vi "Build Weighted Array Histogram.vi"(4 "Reject Negative Weights (T)":bool=TRUE, 5 "Weights":dbl[](array[numeric]), 6 "Data Type (Plot Y Axis)":T4, 7 "Graph Caption (or Label) Text":string, 8 "error in (no error)":errorcluster, 9 "Histogram Options":T1 {"Max Histogram Size" format="%.0e"}, 10 "Plot/Dataset Name":string, 11 "Array":dbl[](array[numeric])) -> (0 "error out":errorcluster, 1 "Message":string, 3 "Data Statistics":dbl[](array[numeric]))   [LabVIEW 2021, in "Histogram Window.lvlib"]
uses:
  Histogram Window.lvlib
  Graphs/Plot Style 3.ctl
  Graphs/Graphs.lvlib
  Plot Histogram.ctl
  Histogram Data Statistics.ctl
  Histogram Window.vi
  Utilities/Utilities.lvlib
  Histogram Window Q Action v2.ctl
  Histogram Window Q Element v2.ctl
  8d0d2780-fcbe-40f9-8a45-ac027e873698.vi
  <userlib>/_OpenG.lib/array/array.llb/openg_array.lvlib
  <userlib>/_OpenG.lib/array/array.llb/Delete Elements from 1D Array (DBL)__ogtk.vi
  <userlib>/_OpenG.lib/array/array.llb/Filter 1D Array (DBL)__ogtk.vi
  Histogram Bin Position.ctl
  Histogram Bin Option.ctl
  Linear Histogram Options.ctl
  Source Data Type.ctl
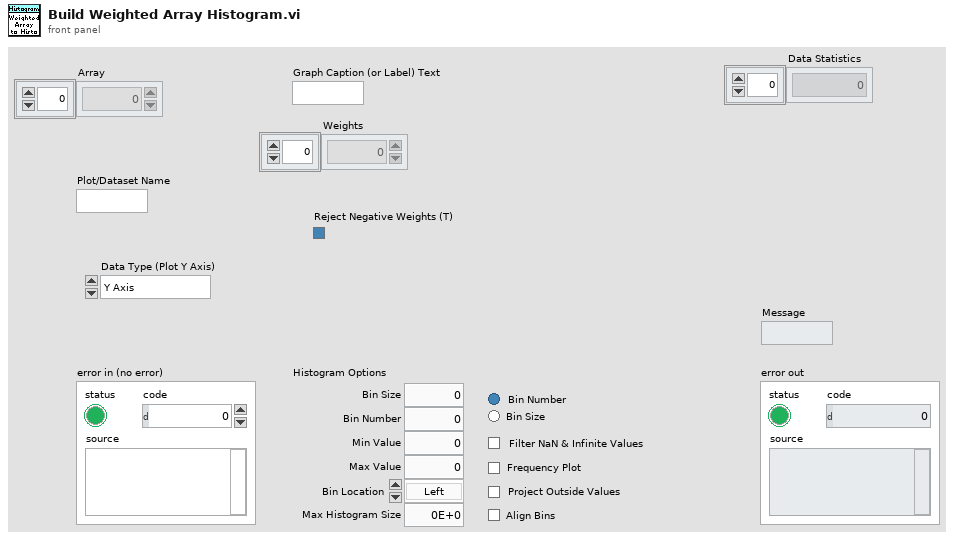
[diagram p1: front panel]
types:
  T1 = typedef "Histogram Window.lvlib/Linear Histogram Options.ctl" = cluster{"Bin Size":dbl, "Bin Number":i32, "Bin Option":T2, "Min Value":dbl, "Max Value":dbl, "Filter NaN & Infinite Values":bool, "Frequency Plot":bool, "Align Bins":bool, "Bin Location":T3, "Project Outside Values":bool, "Max Histogram Size":i32}
  T2 = typedef "Histogram Window.lvlib/Histogram Bin Option.ctl" = enum32{"Bin Number", "Bin Size"}
  T3 = typedef "Histogram Window.lvlib/Histogram Bin Position.ctl" = enum16{"Left", "Center", "Right"}
  T4 = typedef "Histogram Window.lvlib/Source Data Type.ctl" = enum16{"Y Axis", "X Axis", "Single Array"}
  T5 = typedef "Graphs.lvlib/Plot Style 3.ctl" = cluster{"Plot Style":enum16{"unchanged", "Line", "Symbol", "Line + Symbol", "Histogram", "Histogram + Symbol"}, "Histogram Type":enum16{"unchanged", "Left Bound", "Center", "Right Bound"}, "Line Tickness":enum16{"unchanged", "Thin", "1 pixel", "2 pixel", "3 pixel", "4 pixel", "5 pixel"}, "Line Style":enum16{"unchanged", "Plain", "Long Dash", "Short Dash", "Long-Short Dash", "Long-Short-Short Dash"}, "Point Style":enum16{"unchanged", "None", "Empty Circle", "Filled Circle", "Thick Circle", "Dotted Circle", "Empty Square", "Filled Square", "Thick Square", "Dotted Square", "Small Filled Square", "Dot", "Cross", "Tiny Cross", "Large X", "Small x", "Diamond", "Small Empty Square"}, "Line Color":u32, "Point Color":u32, "Anti-aliased":bool, "Line Color Chooser":enum16{"unchanged", "Color Box", "Color List"}, "Point Color Chooser":enum16{"unchanged", "Color Box", "Color List"}, "Line Color List":string, "Point Color List":string}
  T6 = typedef "Histogram Window.lvlib/Histogram Window Q Element v2.ctl" = cluster{"Histogram Window Q Action":T7, "Data":variant}
  T7 = typedef "Histogram Window.lvlib/Histogram Window Q Action v2.ctl" = enum16{"Idle", "Initialization", "Generic XY Graph Event", "Add Histogram", "Delete Plot", "Delete Selected Plots", "Clear Graph", "Change Bin Size", "Invert Histogram", "Update Graph", "Plot Fit", "Export XYGraph to Notebook", "Set Last Cursor Style", "Quit"}
  T8 = typedef "Histogram Window.lvlib/Histogram Data Statistics.ctl" = cluster{"mean":dbl, "standard deviation":dbl, "variance":dbl, "rms value":dbl, "median":dbl, "mode":dbl, "max Value":dbl, "min Value":dbl, "# elements  ":dbl}
  T9 = typedef "Histogram Window.lvlib/Plot Histogram.ctl" = cluster{"Plot Name":string, "Histogram":cluster{"Axis":dbl[], "Histogram":dbl[]}, "Plot Style":T5}
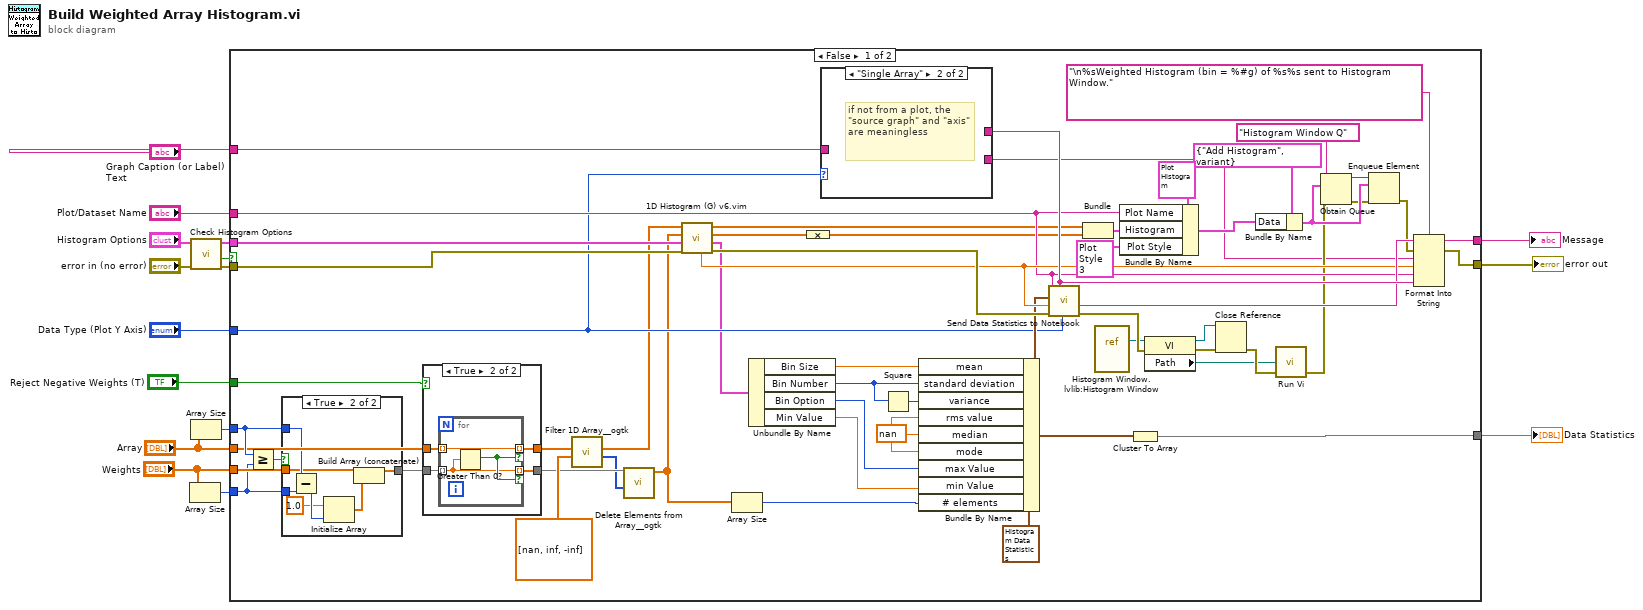
[diagram p0: block diagram]
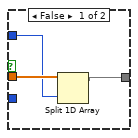
[diagram p3: hidden frame]
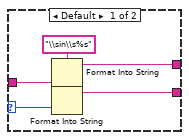
[diagram p4: hidden frame]
diagram:
  n1 = Array Size(array="Weights") -> (size(s)=w2:i32)
  n2 = call "Check Histogram Options.vi"("error in (no error)"="error in (no error)", "Histogram Options in"="Histogram Options") -> ("error out"=w7:errorcluster, "Cancelled?"=w6:bool, "Histogram Options out"=w8:T1)  [unwired: 7 in]
  n3 = Array Size(array="Array") -> (size(s)=w3:i32)
  n4 = case shown="False" w6 {
    tunnel: "Data Type (Plot Y Axis)" -> [w39 _]
    tunnel: "Graph Caption (or Label) Text" -> [w38 _]
    tunnel: "Plot/Dataset Name" -> [w64 _]
    tunnel: [w62 _] -> w13
    tunnel: [w61 w98] -> w12
    tunnel: "Array" -> [w31 _]
    tunnel: [w58 _] -> w11
    tunnel: w8 -> [w41 _]
    tunnel: w7 -> [w40 w98]
    tunnel: "Weights" -> [w35 _]
    tunnel: w3 -> [w34 _]
    tunnel: w2 -> [w33 _]
    tunnel: "Reject Negative Weights (T)" -> [w32 _]
    frame False {
      w21 = nan ("rms value")
      n5 = Greater Or Equal?(x=w34, y=w33) -> (x >= y?=w36:bool)
      n6 = case shown="True" w36 {
        tunnel: w35 -> [w85 w90]
        tunnel: w34 -> [w84 w92]
        tunnel: w33 -> [_ w91]
        tunnel: [w83 w86] -> w30
        frame False {
          n7 = Split 1D Array(array=w85, index=w84) -> (first subarray=w83:dbl[])  [unwired: 1 out]
        }
        frame True {
          n8 = Subtract(x=w92, y=w91) -> (x-y=w89:i32)
          n9 = Initialize Array(1.0 ("element"), w89) -> (w87:dbl[])
          n10 = Build Array (concatenate)(w90, w87) -> (w86:dbl[])
        }
      }
      n11 = case shown="True" w32 {
        tunnel: w31 -> [w75 w79]
        tunnel: w30 -> [w74 w77]
        tunnel: [w75 w78] -> w29
        tunnel: [w74 w76] -> w28
        frame False {
        }
        frame True {
          n12 = for {
            tunnel: w79 -> [w82] mode=indexing
            tunnel: [w82] -> w78 mode=indexing if=w81
            tunnel: w77 -> [w80] mode=indexing
            tunnel: [w80] -> w76 mode=indexing if=w81
            n13 = Greater Than 0?(x=w80) -> (x > 0?=w81:bool)
          }
        }
      }
      n14 = call-poly <userlib>:"Filter 1D Array__ogtk.vi"("items to filter"=dbl[] [nan, inf, -inf] ("Element(s) to Remove"), "array"=w29) -> ("filtered item indices"=w27:i32[], "filtered array"=w25:dbl[])  [unwired: 4 in]
      n15 = call-poly <userlib>:"Delete Elements from Array__ogtk.vi"("indices"=w27, "array"=w28) -> ("array w/ subset deleted"=w24:dbl[])  [unwired: 8 in, 1 out]
      n16 = call "1D Histogram (G) v6.vim"("Error In"=w40, "Histogram Options"=w41, "Weights"=w24, "Array"=w25) -> ("Error Out"=w71:errorcluster, "Histogram Options (out)"=w20:T1, "Histogram"=w48:dbl[], "Axis"=w49:dbl[], "Actual Bin Size"=w70:dbl)  [unwired: 1 in, 2 out]
      n17 = Array Size(array=w24) -> (size(s)=w52:i32)
      n18 = Unbundle By Name(w20) -> ("Bin Size"=w23:dbl, "Bin Number"=w19:i32, "Bin Option"=w18:T2, "Min Value"=w17:dbl)
      n19 = Compound Arithmetic op=MULTIPLY(w48) -> (w26:dbl[])
      n20 = case shown="\"Single Array\"" w39 {
        selector: w39 -> [w94 _]
        tunnel: [w96 _] -> w73
        tunnel: w38 -> [w95 _]
        tunnel: [w93 _] -> w37
        frame Default {
          n21 = Format Into String(format string="\\sin\\s%s", w95) -> (resulting string=w96:string)  [unwired: 2 in, 1 out]
          n22 = Format Into String(w94) -> (resulting string=w93:string)  [unwired: 3 in, 1 out]
        }
        frame "Single Array" {
          # "if not from a plot, the \"source graph\" and \"axis\" are meaningless"
        }
      }
      n23 = Square(x=w19) -> (x^2=w22:i32)
      n24 = Bundle By Name(cluster=T8 {"mean"=0.0, "standard deviation"=0.0, "variance"=0.0, "rms value"=0.0, "median"=0.0, "mode"=0.0, "max Value"=0.0, "min Value"=0.0, "# elements  "=0.0} ("Data Statistics"), "mean"=w23, "standard deviation"=w19, "variance"=w22, "rms value"=w21, "median"=w21, "mode"=w21, "max Value"=w18, "min Value"=w17, "# elements"=w52) -> (w57:T8)
      n25 = call "Send Data Statistics to Notebook.vi"("Source Data Type (Plot Y Axis)"=w39, "Graph Caption"=w73, "Error In"=w71, "Bin"=w70, "Data Statistics"=w57, "Plot/Dataset Name"=w64) -> ("Error Out"=w56:errorcluster, "Message"=w72:string)  [unwired: 4 in]
      n26 = Bundle("Axis"=w49, "Histogram"=w26) -> (w43:cluster{"Axis":dbl[], "Histogram":dbl[]})  [unwired: 1 in]
      n27 = vi-ref "Histogram Window.lvlib:Histogram Window.vi"() -> (w53:refnum<vi>)
      n28 = Bundle By Name(cluster=T9 {"Plot Name"="", "Histogram"={"Axis"=[], "Histogram"=[]}, "Plot Style"={"Plot Style"=enum."Histogram + Symbol", "Histogram Type"=enum."Right Bound", "Line Tickness"=enum."unchanged", "Line Style"=enum."unchanged", "Point Style"=enum."unchanged", "Line Color"=0, "Point Color"=0, "Anti-aliased"=FALSE, "Line Color Chooser"=enum."unchanged", "Point Color Chooser"=enum."unchanged", "Line Color List"="", "Point Color List"=""}} ("output cluster"), "Plot Name"=w64, "Histogram"=w43, "Plot Style"=T5 {"Plot Style"=enum."Histogram", "Histogram Type"=enum."Left Bound", "Line Tickness"=enum."1 pixel", "Line Style"=enum."Plain", "Point Style"=enum."None", "Line Color"=0, "Point Color"=0, "Anti-aliased"=TRUE, "Line Color Chooser"=enum."Color Box", "Point Color Chooser"=enum."unchanged", "Line Color List"="", "Point Color List"=""}) -> (w47:T9)
      n29 = Cluster To Array(cluster=w57) -> (array=w58:dbl[])
      n30 = property class="VI"(reference=w53, error in=w56) -> (reference out=w54:refnum<vi>, error out=w68:errorcluster, "Path"=w55:path)
      n31 = Close Reference(reference=w54, error in (no error)=w68) -> (error out=w69:errorcluster)
      n32 = Bundle By Name(cluster=T6 {"Histogram Window Q Action"=enum."Add Histogram", "Data"=variant} ("ALEX TT Histogram Q Element"), "Data"=w47) -> (w66:T6)
      n33 = call "Run Vi.vi"("VI Path"=w55, "error in (no error)"=w69) -> ("error out"=w50:errorcluster)  [unwired: 6 in, 1 out]
      n34 = Obtain Queue(name (unnamed)="Histogram Window Q", element data type=w66, error in (no error)=w50) -> (queue out=w44:refnum<queue>, error out=w46:errorcluster)  [unwired: 2 in, 1 out]
      n35 = Enqueue Element(queue=w44, element=w66, error in (no error)=w46) -> (error out=w60:errorcluster)  [unwired: 1 in, 2 out]
      n36 = Format Into String(format string="\n%sWeighted Histogram (bin = %#g) of %s%s sent to Histogram Window.", initial string=w72, error in=w60, w37, w70, w64, w73) -> (resulting string=w62:string, error out=w61:errorcluster)
    }
    frame True {
    }
  }
  "Message" <- w13
  "error out" <- w12
  "Data Statistics" <- w11
